vi "Hatch Teleop.vi"(6 "Auto Align":bool, 10 "POV Value":i16, 11 "Hatch toggle":bool) -> ()   [LabVIEW 2018]
uses:
  Implementation/Hatch Intake Published Globals.vi
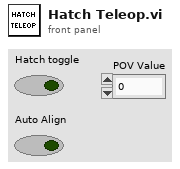
[diagram p1: front panel]
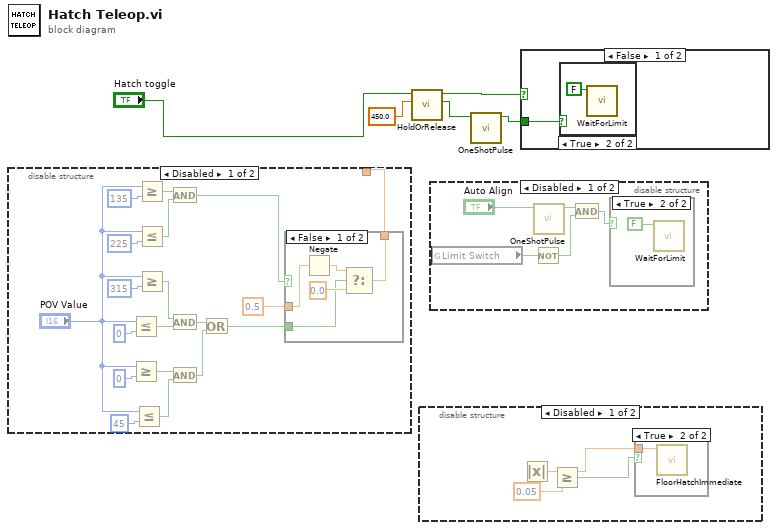
[diagram p0: block diagram]
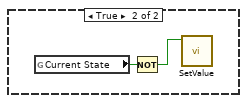
[diagram p3: hidden frame]
diagram:
  n1 = disable-structure shown="Disabled" {
    disable-tunnel: [w8 _] -> _
    frame Disabled {
      n2 = Less Or Equal?(x="POV Value", y=0) -> (x <= y?=w18:bool)
      n3 = Greater Or Equal?(x="POV Value", y=0) -> (x >= y?=w11:bool)
      n4 = Less Or Equal?(x="POV Value", y=45) -> (x <= y?=w12:bool)
      n5 = Greater Or Equal?(x="POV Value", y=135) -> (x >= y?=w22:bool)
      n6 = Less Or Equal?(x="POV Value", y=225) -> (x <= y?=w21:bool)
      n7 = Greater Or Equal?(x="POV Value", y=315) -> (x >= y?=w17:bool)
      n8 = And(x=w22, y=w21) -> (x .and. y?=w9:bool)
      n9 = And(x=w17, y=w18) -> (x .and. y?=w16:bool)
      n10 = And(x=w11, y=w12) -> (x .and. y?=w10:bool)
      n11 = Or(x=w16, y=w10) -> (x .or. y?=w6:bool)
      n12 = case shown="False" w9 {
        tunnel: [w25 w30] -> w8
        tunnel: 0.5 -> [w27 w30]
        tunnel: w6 -> [w26 _]
        frame False {
          n13 = Negate(x=w27) -> (-x=w28:dbl)
          n14 = Select(t=w28, s=w26, f=0.0) -> (s? t:f=w25:dbl)
        }
        frame True {
        }
      }
    }
    frame Enabled {
    }
  }
  n15 = call "HoldOrRelease.vi"("Delay"=450.0, "Right Bumper"="Hatch toggle") -> ("Call Auto-Hatch"=w2:bool, "Call Toggle"=w3:bool)  [unwired: 8 in]
  n16 = disable-structure shown="Disabled" {
    frame Disabled {
      n17 = Absolute Value(x=w33) -> (abs(x)=w34:dbl)
      n18 = Greater Or Equal?(x=w34, y=0.05) -> (x >= y?=w31:bool)
      n19 = case shown="True" w31 {
        tunnel: [_ w35] -> w33
        frame False {
        }
        frame True {
          n20 = call "FloorHatchImmediate.vi"("Speed"=w35) -> ()  [unwired: 10 in, 1 out]
        }
      }
    }
    frame Enabled {
    }
  }
  n21 = disable-structure shown="Disabled" {
    frame Disabled {
      n22 = global read "Hatch Intake Published Globals.vi" "Limit Switch"() -> (w37:bool)
      n23 = Not(x=w37) -> (.not. x?=w36:bool)
      n24 = call "OneShotPulse.vi"("Input"="Auto Align") -> ("Output"=w39:bool)  [unwired: 10 in]
      n25 = And(x=w39, y=w36) -> (x .and. y?=w38:bool)
      n26 = case shown="True" w38 {
        frame False {
        }
        frame True {
          n27 = call "WaitForLimit.vi"("Value"=FALSE) -> ()  [unwired: 10 in, 1 out]
        }
      }
    }
    frame Enabled {
    }
  }
  n28 = call "OneShotPulse.vi"("Input"=w2) -> ("Output"=w1:bool)  [unwired: 10 in]
  n29 = case shown="False" w3 {
    tunnel: w1 -> [w42 _]
    frame False {
      n30 = case shown="True" w42 {
        frame False {
        }
        frame True {
          n31 = call "WaitForLimit.vi"("Value"=FALSE) -> ()  [unwired: 10 in, 1 out]
        }
      }
    }
    frame True {
      n32 = global read "Hatch Intake Published Globals.vi" "Current State"() -> (w45:bool)
      n33 = Not(x=w45) -> (.not. x?=w44:bool)
      n34 = call "SetValue.vi"("Value"=w44) -> ()  [unwired: 10 in, 1 out]
    }
  }
